vi "setLUT.vi"(0 "HGF_IMAQDevice in":refnum<class "HGF_IMAQDevice.lvclass">, 1 "Tap 0 LUT (Red)":u16[](array[numeric]), 2 "Tap 1 LUT (Green)":u16[](array[numeric]), 3 "Tap 2 LUT (Blue)":u16[](array[numeric]), 4 "Tap 3 LUT":u16[](array[numeric]), 5 "error in (no error)":errorcluster) -> (14 "HGF_IMAQDevice out":refnum<class "HGF_IMAQDevice.lvclass">, 19 "error out":errorcluster)   [LabVIEW 2014, in "HGF_IMAQ.lvlib" / "HGF_IMAQDevice.lvclass"]
doc: "Downloads a custom lookup table (LUT) to an image acquisition device. This VI can download 8-bit or 16-bit LUTs for analog or digital devices. If the image acquisition device has multiple LUTs, you can input all of the LUTs into this VI. Call this VI before starting the acquisition."
uses:
  HGF_IMAQDevice.lvclass
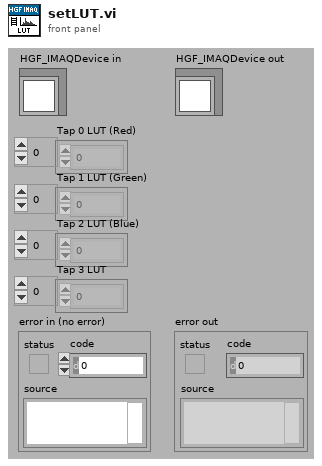
[diagram p1: front panel]
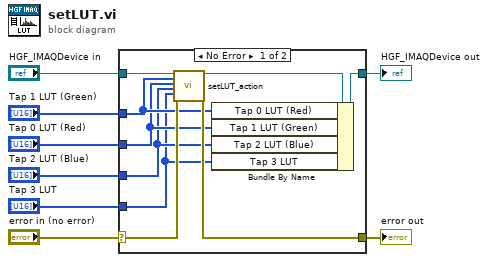
[diagram p0: block diagram]
diagram:
  n1 = case shown="No Error" "error in (no error)" {
    selector: "error in (no error)" -> [w17 w19]
    tunnel: [w16 w19] -> w7
    tunnel: [w9 w18] -> w5
    tunnel: "HGF_IMAQDevice in" -> [w15 w18]
    tunnel: "Tap 1 LUT (Green)" -> [w14 _]
    tunnel: "Tap 0 LUT (Red)" -> [w13 _]
    tunnel: "Tap 2 LUT (Blue)" -> [w12 _]
    tunnel: "Tap 3 LUT" -> [w11 _]
    frame No Error {
      n2 = call-dynamic "setLUT_action.vi"("HGF_IMAQDevice in"=w15, "Tap 0 LUT (Red)"=w14, "Tap 1 LUT (Green)"=w13, "Tap 2 LUT (Blue)"=w12, "Tap 3 LUT"=w11, "error in (no error)"=w17) -> ("HGF_IMAQDevice out"=w10:refnum<class "HGF_IMAQDevice.lvclass">, "error out"=w16:errorcluster)  [unwired: 12 in]
      n3 = Bundle By Name(cluster=w10, "Tap 0 LUT (Red)"=w14, "Tap 1 LUT (Green)"=w13, "Tap 2 LUT (Blue)"=w12, "Tap 3 LUT"=w11) -> (w9:refnum<class "HGF_IMAQDevice.lvclass">)
    }
    frame Error {
    }
  }
  "error out" <- w7
  "HGF_IMAQDevice out" <- w5
